vi "Init.vi"(8 "error in (no error)":errorcluster) -> (0 "error out":errorcluster, 3 "VMR Server out":refnum<class "VMR Server.lvclass">)   [LabVIEW 2022 SP3, in "VMR Server.lvlib" / "VMR Server.lvclass"]
uses:
  VMR Server.lvclass
  VMR Server.lvclass/VMR Server.ctl
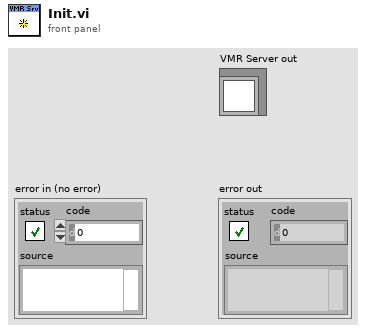
[diagram p1: front panel]
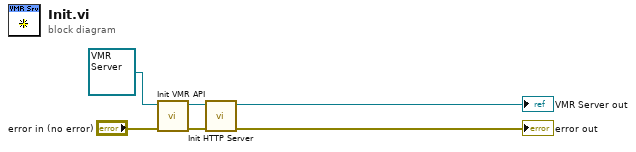
[diagram p0: block diagram]
diagram:
  n1 = call "Init VMR API.vi"("error in (no error)"="error in (no error)", "VMR Server in"=refnum<class "VMR Server.lvclass"> refnum) -> ("error out"=w5:errorcluster, "VMR Server out"=w2:refnum<class "VMR Server.lvclass">)  [unwired: 8 in]
  n2 = call "Init HTTP Server.vi"("error in (no error)"=w5, "VMR Server in"=w2) -> ("error out"=→"error out":errorcluster, "VMR Server out"=→"VMR Server out":refnum<class "VMR Server.lvclass">)  [unwired: 8 in]
